vi "Create RND Tour.vi"(11 "City's":u16=3) -> (3 "Tour":u16[](array[numeric])=[1, 14, 13, 12, 7, 6, 15, 5, 11, 9, 10, 16, 3, 2, 4, 8, 1])   [LabVIEW 2015, in "TSP Library.lvlib"]
uses:
  TSP Library.lvlib
  <vilib>/Analysis/1siggen.llb/Ramp Pattern by Delta.vi
  <vilib>/Analysis/NI_AALBase.lvlib
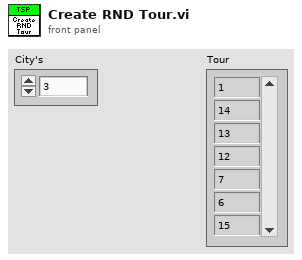
[diagram p1: front panel]
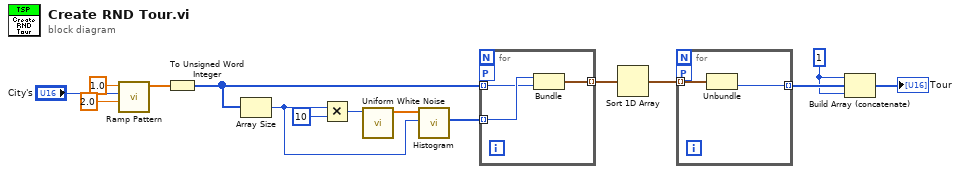
[diagram p0: block diagram]
diagram:
  w1 = u16 1
  n1 = call-poly <vilib>:"Ramp Pattern.vi"("start"=2.0, "end"="City's", "delta"=1.0) -> ("Ramp Pattern"=w5:dbl[])  [unwired: 6 in, 2 out]
  n2 = To Unsigned Word Integer(number=w5) -> (unsigned 16bit integer=w4:u16[])
  n3 = Array Size(array=w4) -> (size(s)=w12:i32)
  n4 = Multiply(x=w12, y=10) -> (x*y=w14:i32)
  n5 = call <vilib>:"Uniform White Noise.vi"("samples"=w14) -> ("uniform white noise"=w13:dbl[])  [unwired: 9 in, 1 out]
  n6 = call <vilib>:"Histogram.vi"("intervals"=w12, "X"=w13) -> ("Histogram: h(x)"=w11:i32[])  [unwired: 6 in, 3 out]
  n7 = for {
    tunnel: w4 -> [w17] mode=indexing
    tunnel: w11 -> [w18] mode=indexing
    tunnel: [w16] -> w10 mode=indexing
    workers-P: _ -> [_]
    n8 = Bundle(w18, w17) -> (w16:cluster{i32, u16})  [unwired: 1 in]
  }
  n9 = Sort 1D Array(array=w10) -> (sorted array=w9:cluster{i32, u16}[])
  n10 = for {
    tunnel: w9 -> [w20] mode=indexing
    tunnel: [w19] -> w3 mode=indexing
    workers-P: _ -> [_]
    n11 = Unbundle(w20) -> (w19:u16)  [unwired: 1 out]
  }
  n12 = Build Array (concatenate)(w1, w3, w1) -> (→"Tour":u16[])
